vi "Chassis3FPGA.vi"() -> ()   [LabVIEW 2018]
uses:
  <vilib>/rvi/Emulation/niFpgaGetClockAttributes.vi
  <vilib>/rvi/Emulation/niFpgaSctlEmulationGetInTimedLoop.vi
  <vilib>/rvi/Emulation/niFpgaEmulationReportErrorSimple.vi
  <vilib>/rvi/eio/common/nirviEmuTemplateMethod_errors.vi
  <vilib>/rvi/Emulation/niFpgaProcessEmulError.vi
  <vilib>/rvi/Emulation/niFpgaCriticalErrorInLSC.vi
  <vilib>/rvi/eio/common/nirviEmuTemplatePropertyGet_errors.vi
  <vilib>/rvi/interface/RandomDataEmulation/niFpgaRandomDataHandleErrors.vi
  <vilib>/eio/EIOMethodNode/EIOMethodNode.xnode
  <vilib>/eio/EIONode/EIONode.xnode
  <vilib>/eio/EIOPropertyNode/EIOPropertyNode.xnode
  <vilib>/rvi/DataTransferAndStorage/Container/XNode/niFpgaContainer.xnode
  <vilib>/rvi/interface/RandomDataEmulation/nirviRandomDataFpgaReadWriteTemplate.vi
  <vilib>/rvi/eio/common/nirviEmuTemplatePropertyGet_noerrors.vi
  <vilib>/rvi/eio/common/nirviEmuTemplatePropertySet_errors.vi
  <vilib>/rvi/eio/common/nirviEmuTemplatePropertySet_noerrors.vi
panel:
  in  "Label Filter":T1
  out "Rx Status":u16 format="%016b"
  in  "Rx Channel Number":u8 max=7 step=1
  in  "Rx Config Data (RCR)":u16=33 format="%04x"
  in  "Tx Data":u32=305419896 format="%08x"
  in  "Transmit Data":bool
  in  "Tx Config Data (TCR)":u16=8192 format="%04x"
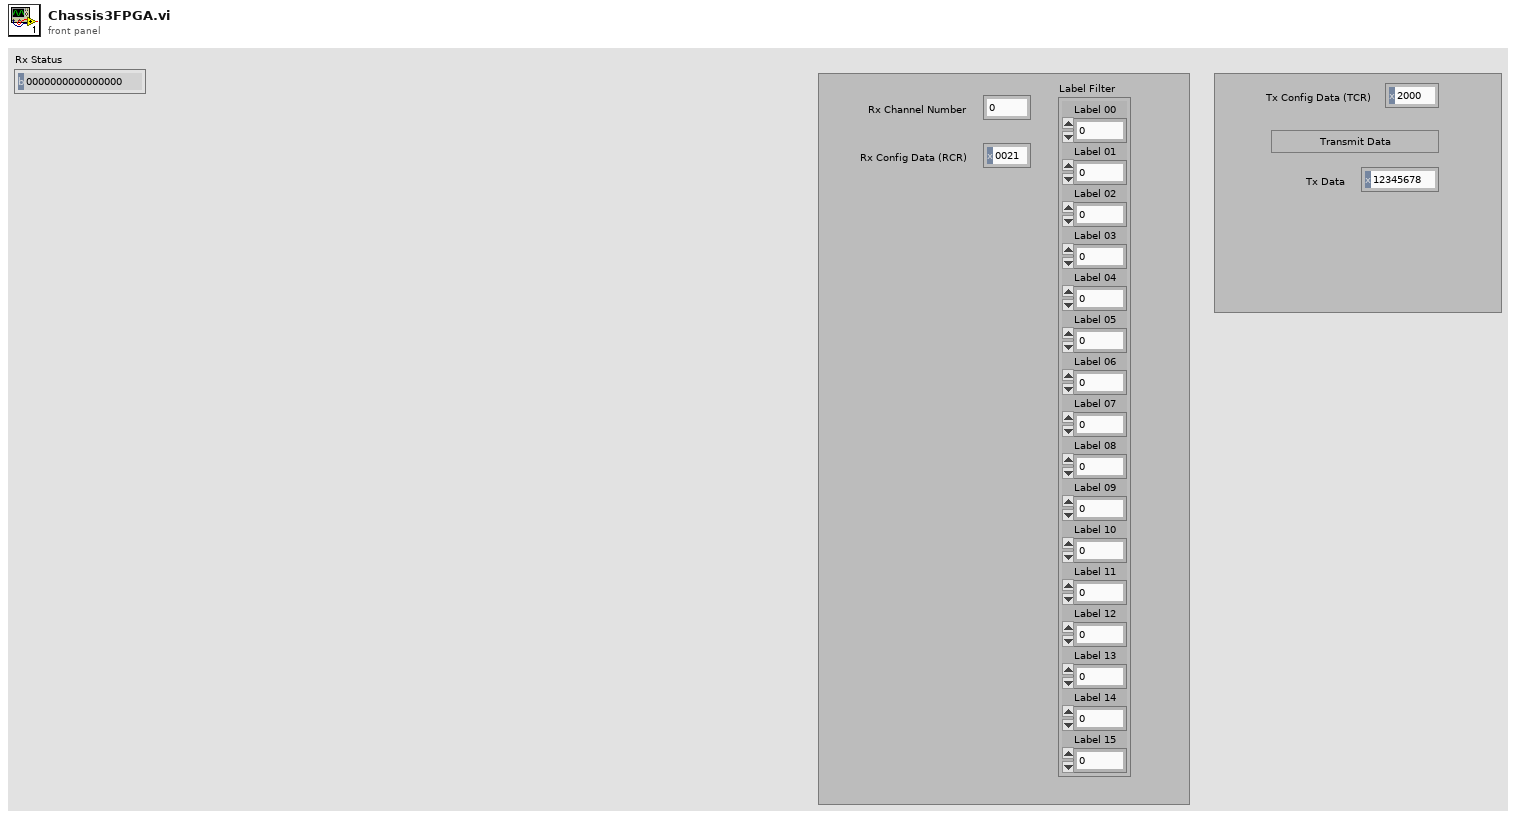
[diagram p1: front panel]
types:
  T1 = cluster{"Label 00":u8, "Label 01":u8, "Label 02":u8, "Label 03":u8, "Label 04":u8, "Label 05":u8, "Label 06":u8, "Label 07":u8, "Label 08":u8, "Label 09":u8, "Label 10":u8, "Label 11":u8, "Label 12":u8, "Label 13":u8, "Label 14":u8, "Label 15":u8}
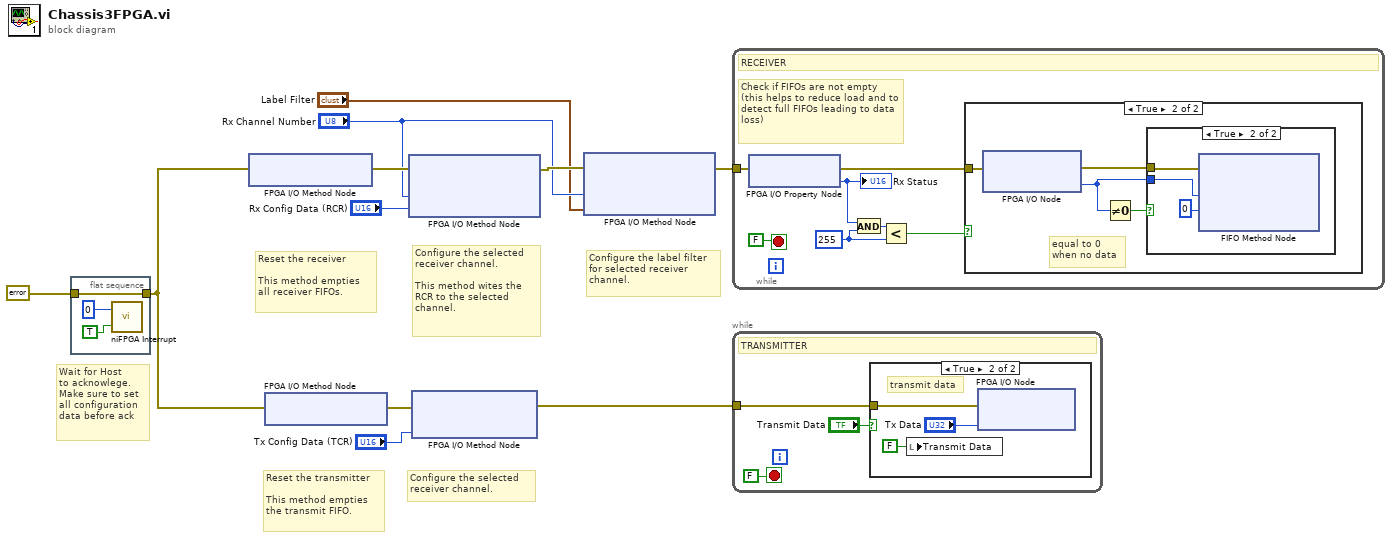
[diagram p0: block diagram]
diagram:
  # "Configure the label filter\nfor selected receiver\nchannel."
  # "Wait for Host\nto acknowlege.\nMake sure to set \nall configuration\ndata before ack"
  # "Configure the selected\nreceiver channel."
  # "Reset the transmitter\n\nThis method empties\nthe transmit FIFO."
  # "Configure the selected\nreceiver channel.\n\nThis method wites the\nRCR to the selected\nchannel."
  # "Reset the receiver\n\nThis method empties\nall receiver FIFOs."
  n1 = flat-sequence {
    tunnel: errorcluster {"status"=FALSE, "code"=0, "source"=""} ("error out") -> [w12]
    tunnel: [w12] -> w5
    frame #0 {
      n2 = call <vilib>:"niFPGA Interrupt.vi"("Wait Until Cleared (F)"=TRUE ("Wait Until Cleared"), "IRQ Number (0)"=u8 0 ("IRQ Bit (0-31)")) -> ()  [unwired: 1 in]
    }
  }
  n3 = xnode "FPGA I/O Method Node"("error in"=w5) -> ("error out"=w9:errorcluster)  [unwired: 1 in, 1 out]
  n4 = xnode "FPGA I/O Method Node"("error in"=w5) -> ("error out"=w8:errorcluster)  [unwired: 1 in, 1 out]
  n5 = xnode "FPGA I/O Method Node"("error in"=w9, "Channel Number"="Rx Channel Number", "Control Register"="Rx Config Data (RCR)") -> ("error out"=w4:errorcluster)  [unwired: 1 in, 1 out]
  n6 = xnode "FPGA I/O Method Node"("error in"=w8, "Control Register"="Tx Config Data (TCR)") -> ("error out"=w7:errorcluster)  [unwired: 1 in, 1 out]
  n7 = xnode "FPGA I/O Method Node"("error in"=w4, "Channel Number"="Rx Channel Number", "Label Filter"="Label Filter") -> ("error out"=w3:errorcluster)  [unwired: 1 in, 1 out]
  n8 = while {
    tunnel: w3 -> [w17]
    stop <- FALSE stop-if-true
    w18 = u16 255 ("y")
    # "Check if FIFOs are not empty\n(this helps to reduce load and to detect full FIFOs leading to data loss)"
    # "RECEIVER"
    n9 = xnode "FPGA I/O Property Node"("error in"=w17) -> ("error out"=w15:errorcluster, "Rx Status"=w19:u16)  [unwired: 1 in, 1 out]
    "Rx Status" <- w19
    n10 = And(x=w19, y=w18) -> (x .and. y?=w20:u16)
    n11 = Less?(x=w20, y=w18) -> (x < y?=w16:bool)
    n12 = case shown="True" w16 {
      tunnel: w15 -> [_ w22]
      frame False {
      }
      frame True {
        # "equal to 0\nwhen no data"
        n13 = xnode "FPGA I/O Node"("error in"=w22) -> ("error out"=w23:errorcluster, "Mod8/Rx0"=w25:u32)  [unwired: 1 in, 1 out]
        n14 = Not Equal To 0?(x=w25) -> (x != 0?=w24:bool)
        n15 = case shown="True" w24 {
          tunnel: w25 -> [_ w28]
          tunnel: w23 -> [_ w26]
          frame False {
          }
          frame True {
            n16 = xnode ("FIFO Method Node")("Element"=w28, "Timeout"=0, "error in (no error)"=w26) -> ()  [unwired: 1 in, 3 out]
          }
        }
      }
    }
  }
  n17 = while {
    tunnel: w7 -> [w29]
    stop <- FALSE stop-if-true
    # "TRANSMITTER"
    n18 = case shown="True" "Transmit Data" {
      tunnel: w29 -> [_ w32]
      frame False {
      }
      frame True {
        # "transmit data"
        n19 = local write "Transmit Data"(FALSE ("Transmit Data")) -> ()
        n20 = xnode "FPGA I/O Node"("error in"=w32, "Mod8/Tx0"="Tx Data") -> ()  [unwired: 1 in, 2 out]
      }
    }
  }
